vi "midi_ParseTracks.vi"(8 "error in (no error)":errorcluster, 10 "header info":T2, 11 "string in":string) -> (0 "error out":errorcluster, 3 "file contents":T1)   [LabVIEW 2013]
doc: "Parse the tracks of a standard MIDI file."
panel:
  # "midi_ParseTracks.vi"
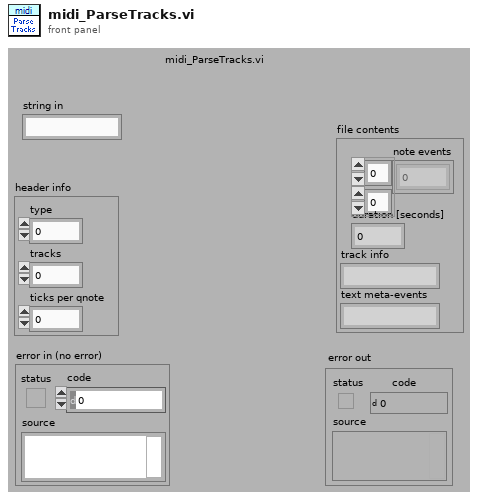
[diagram p1: front panel]
types:
  T1 = cluster{"note events":dbl[][], "duration [seconds]":dbl, "track info":string, "text meta-events":string}
  T2 = cluster{"type":u16, "tracks":u16, "ticks per qnote":u16}
  T3 = cluster{"status":u8, "channel":u8, "data byte 1":u8, "data byte 2":u8, "tempo":u32, "track name":string, "text":string}
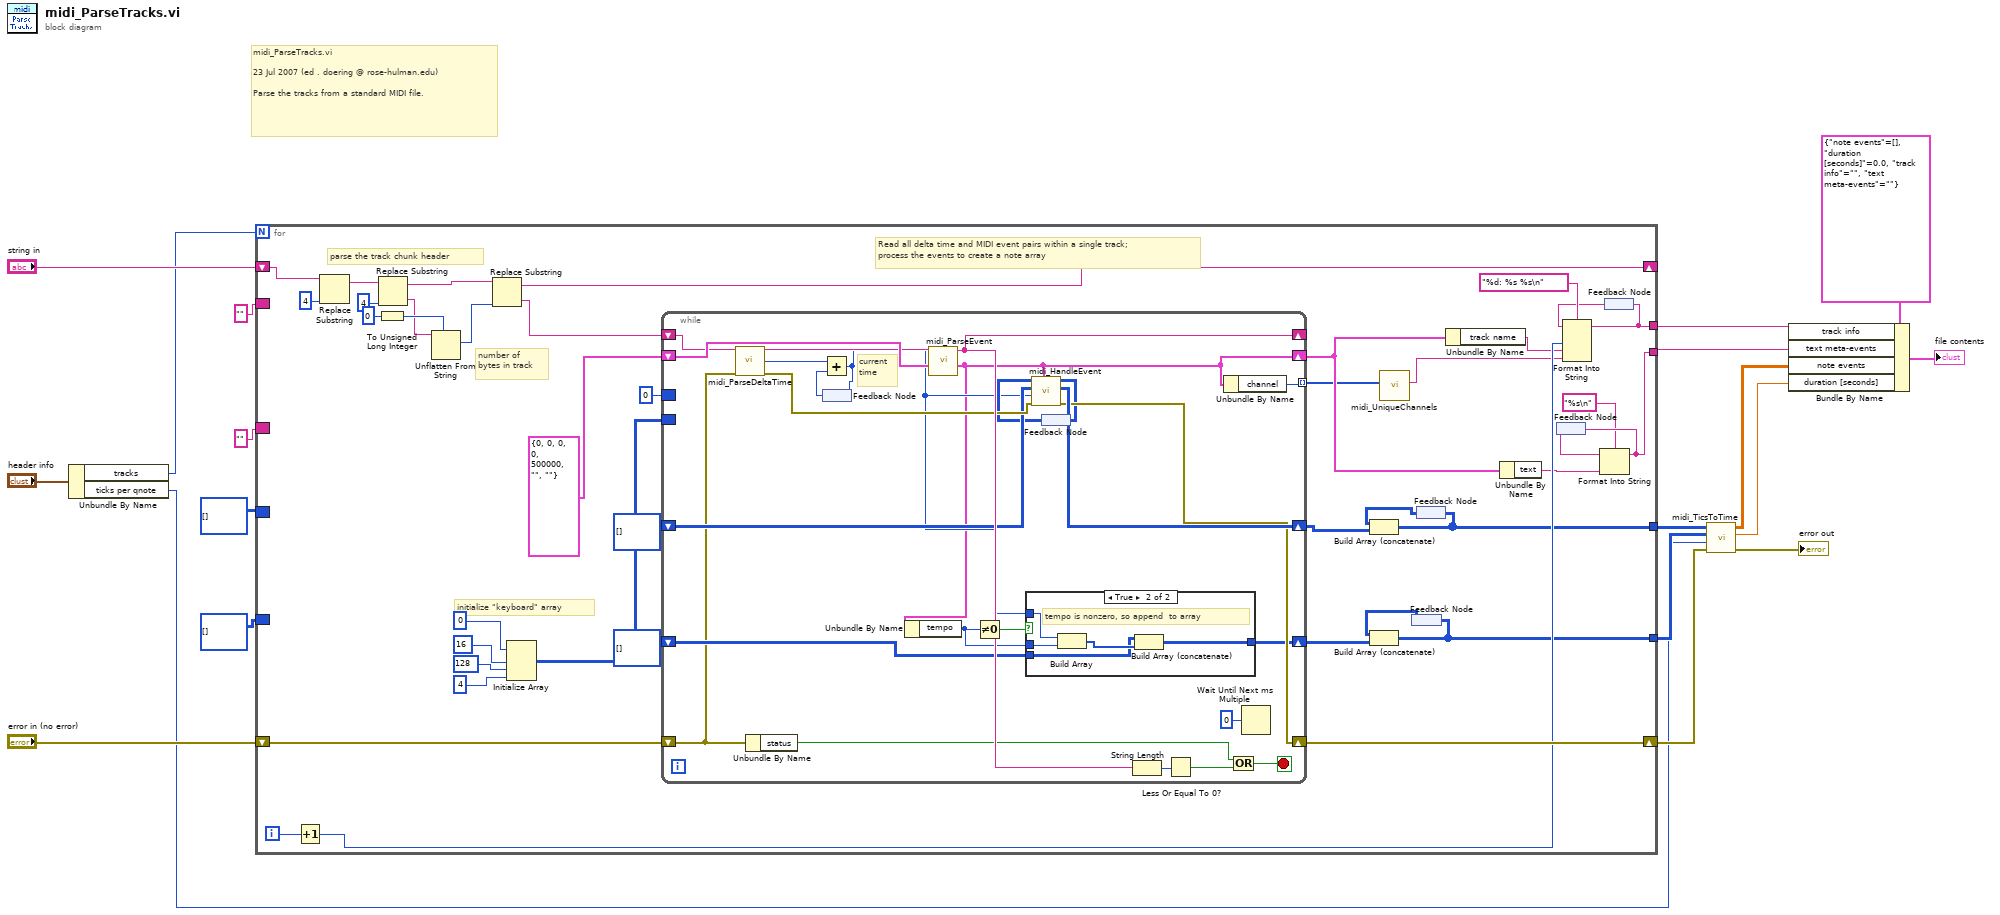
[diagram p0: block diagram]
diagram:
  # "midi_ParseTracks.vi\n\n23 Jul 2007 (ed . doering @ rose-hulman.edu)\n\nParse the tracks from a standard MIDI file."
  n1 = Unbundle By Name("header info") -> ("tracks"=w8:u16, "ticks per qnote"=w7:u16)
  n2 = for {
    N: w8 -> [_]
    shift-right: [w41] -> _
    shift-left: "string in" -> [w54]
    shift-right: [w43] -> w15
    shift-left: "error in (no error)" -> [w44]
    tunnel: [w36] -> w5
    tunnel: [w34] -> w4
    tunnel: [w27] -> w12
    tunnel: [w25] -> w11
    border: "" -> [_]
    border: "" -> [_]
    border: u32[][] [] -> [_]
    border: u32[][] [] -> [_]
    i -> [w20]
    # "number of\nbytes in track"
    # "parse the track chunk header"
    # "initialize \"keyboard\" array"
    # "Read all delta time and MIDI event pairs within a single track;\nprocess the events to create a note array"
    n3 = Increment(x=w20) -> (x+1=w39:i32)
    n4 = Replace Substring(2:4 ("length (len. of substring)"), 5:w54) -> (1:w55:string)  [unwired: 2 in, 1 out]
    n5 = To Unsigned Long Integer(number=u32 0) -> (unsigned 32bit integer=w59:u32)
    n6 = Replace Substring(2:4 ("length (len. of substring)"), 5:w55) -> (0:w52:string, 1:w53:string)  [unwired: 2 in]
    n7 = Unflatten From String(type=w59, binary string=w52) -> (value=w58:u32)  [unwired: 3 in, 2 out]
    n8 = Replace Substring(2:w58, 5:w53) -> (0:w42:string, 1:w41:string)  [unwired: 2 in]
    n9 = Initialize Array(u32 0 ("element"), 16 ("dimension size"), 128 ("dimension size"), 4 ("dimension size")) -> (w30:u32[][][])
    n10 = while {
      shift-right: [w66] -> w45
      shift-left: T3 {"status"=0, "channel"=0, "data byte 1"=0, "data byte 2"=0, "tempo"=500000, "track name"="", "text"=""} ("output cluster") -> [w85]
      shift-right: [w84] -> _
      shift-left: w42 -> [w81]
      shift-right: [w77] -> w43
      shift-left: w44 -> [w65]
      tunnel: [w79] -> w21 mode=indexing
      shift-right: [w83] -> w46
      shift-left: u32[][] [] ("note out") -> [w74]
      shift-right: [w68] -> w24
      shift-left: u32[][] [] -> [w67]
      border: u32 0 -> [_]
      border: w30 -> [_]
      stop <- w64 stop-if-true
      # "current\ntime"
      n11 = call "midi_ParseDeltaTime.vi"("string"=w81, "error in (no error)"=w65) -> ("result string"=w82:string, "delta time (tics)"=w76:u32, "error out"=w78:errorcluster)  [unwired: 10 in, 1 out]
      n12 = Unbundle By Name(w65) -> ("status"=w62:bool)
      n13 = feedback #1() -> (w75:u32)
      n14 = Add(x=w76, y=w75) -> (x+y=w69:u32)
      n15 = feedback-in #1(w69) -> ()
      n16 = call "midi_ParseEvent.vi"("input cluster"=w85, "string"=w82) -> ("output cluster"=w66:T3, "result string"=w84:string)  [unwired: 8 in]
      n17 = Unbundle By Name(w66) -> ("tempo"=w70:u32)
      n18 = Not Equal To 0?(x=w70) -> (x != 0?=w71:bool)
      n19 = case shown="True" w71 {
        tunnel: w70 -> [_ w91]
        tunnel: w69 -> [_ w90]
        tunnel: [w86 w88] -> w68
        tunnel: w67 -> [w86 w87]
        frame False {
          # "tempo is zero, so pass the\narray through unchanged"
        }
        frame True {
          # "tempo is nonzero, so append  to array"
          n20 = Build Array(w90, w91) -> (w89:u32[])
          n21 = Build Array (concatenate)(w87, w89) -> (w88:u32[][])
        }
      }
      n22 = feedback #2() -> (w72:u32[][][])
      n23 = call "midi_HandleEvent.vi"("event"=w66, "error in (no error)"=w78, "current time (tics)"=w69, "note in"=w74, "keyboard in"=w72) -> ("error out"=w77:errorcluster, "note out"=w83:u32[][], "keyboard out"=w73:u32[][][])  [unwired: 4 in]
      n24 = feedback-in #2(w73) -> ()
      n25 = String Length(string=w84) -> (length=w80:i32)
      n26 = Less Or Equal To 0?(x=w80) -> (x <= 0?=w63:bool)
      n27 = Unbundle By Name(w66) -> ("channel"=w79:u8)
      n28 = Or(x=w62, y=w63) -> (x .or. y?=w64:bool)
      n29 = Wait Until Next ms Multiple(millisecond multiple=u32 0) -> ()  [unwired: 1 out]
    }
    n30 = call "midi_UniqueChannels.vi"("channels"=w21) -> ("channel list"=w22:string)  [unwired: 10 in]
    n31 = feedback #3() -> (w26:u32[][])
    n32 = Build Array (concatenate)(w26, w24) -> (w25:u32[][])
    n33 = feedback-in #3(w25) -> ()
    n34 = feedback #4() -> (w28:u32[][])
    n35 = Build Array (concatenate)(w28, w46) -> (w27:u32[][])
    n36 = feedback-in #4(w27) -> ()
    n37 = Unbundle By Name(w45) -> ("track name"=w38:string)
    n38 = Unbundle By Name(w45) -> ("text"=w35:string)
    n39 = feedback #5() -> (w33:string)
    n40 = Format Into String(format string="%s\n", initial string=w33, w35) -> (resulting string=w34:string)  [unwired: 1 in, 1 out]
    n41 = feedback-in #5(w34) -> ()
    n42 = feedback #6() -> (w37:string)
    n43 = Format Into String(format string="%d: %s %s\n", initial string=w37, w39, w38, w22) -> (resulting string=w36:string)  [unwired: 1 in, 1 out]
    n44 = feedback-in #6(w36) -> ()
  }
  n45 = call "midi_TicsToTime.vi"("error in (no error)"=w15, "ticks per qnote"=w7, "tempo"=w11, "notes in"=w12) -> ("error out"=→"error out":errorcluster, "duration (s)"=w2:dbl, "notes out"=w3:dbl[][])  [unwired: 5 in]
  n46 = Bundle By Name(cluster=T1 {"note events"=[], "duration [seconds]"=0.0, "track info"="", "text meta-events"=""}, "track info"=w5, "text meta-events"=w4, "note events"=w3, "duration [seconds]"=w2) -> (→"file contents":T1)
